vi "DAQ_Analog_Read.vi"(8 "error in (no error)":errorcluster, 11 "task/channels in":refnum<k21>="Photodetectors") -> (0 "error out":errorcluster, 2 "output cluster":T1, 3 "task out":refnum<k21>)   [LabVIEW 2018]
uses:
  SupportVIs/DAQmx Read (Analog 1D DBL NChan 1Samp).vi
  SupportVIs/DAQmx Fill In Error Info.vi
  SupportVIs/NI_PtbyPt.lvlib
panel:
  out "Waveform Chart - Light":T2(graph)
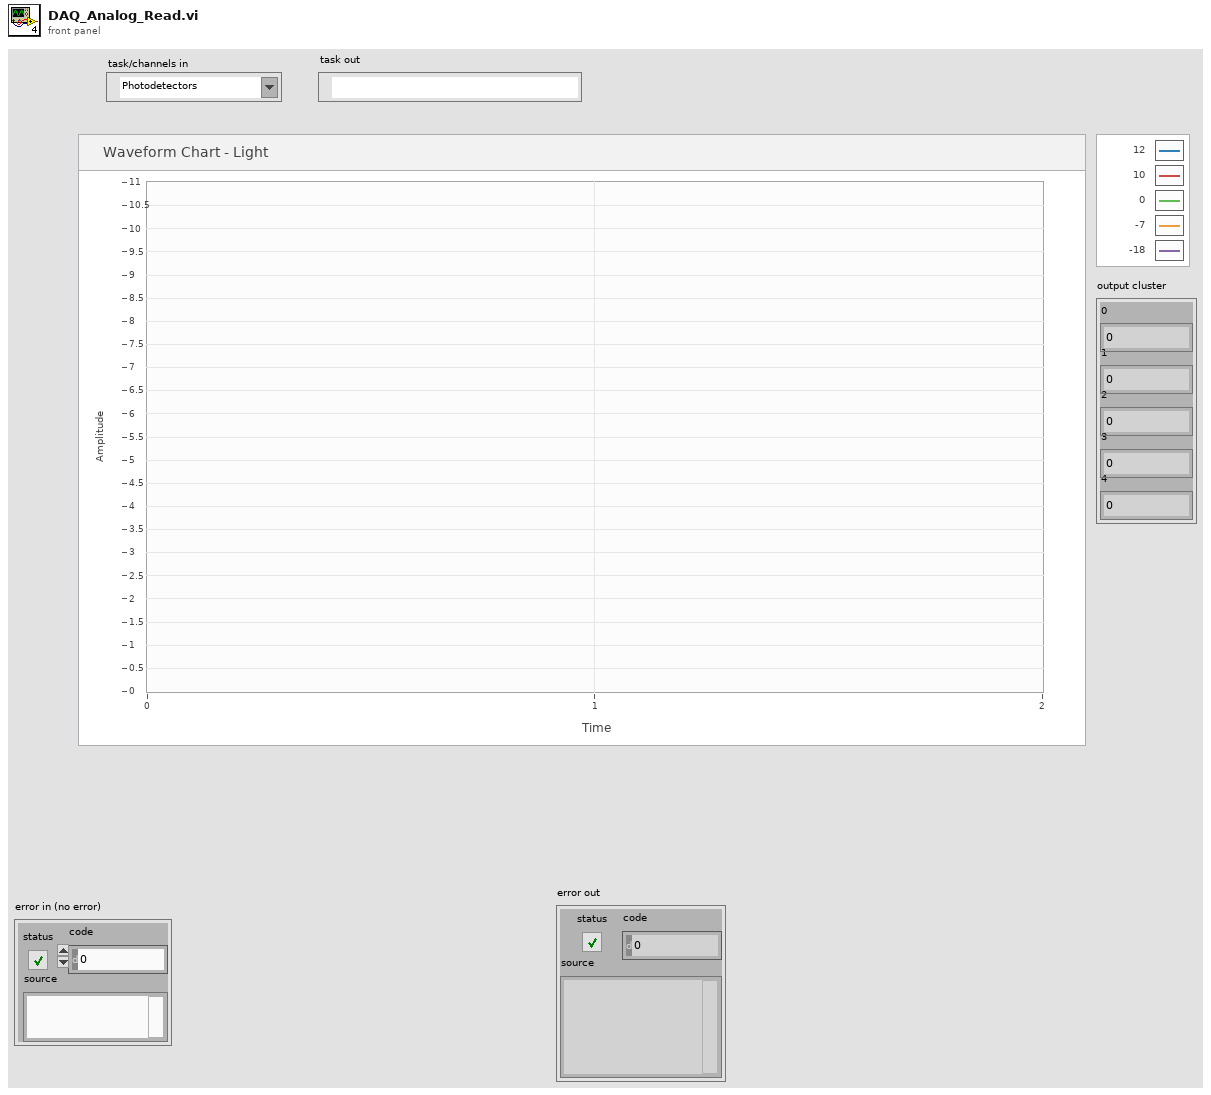
[diagram p1: front panel]
types:
  T1 = cluster{"0":dbl, "1":dbl, "2":dbl, "3":dbl, "4":dbl}
  T2 = cluster{"mean":dbl, "mean":dbl, "mean":dbl, "mean":dbl, "mean":dbl}
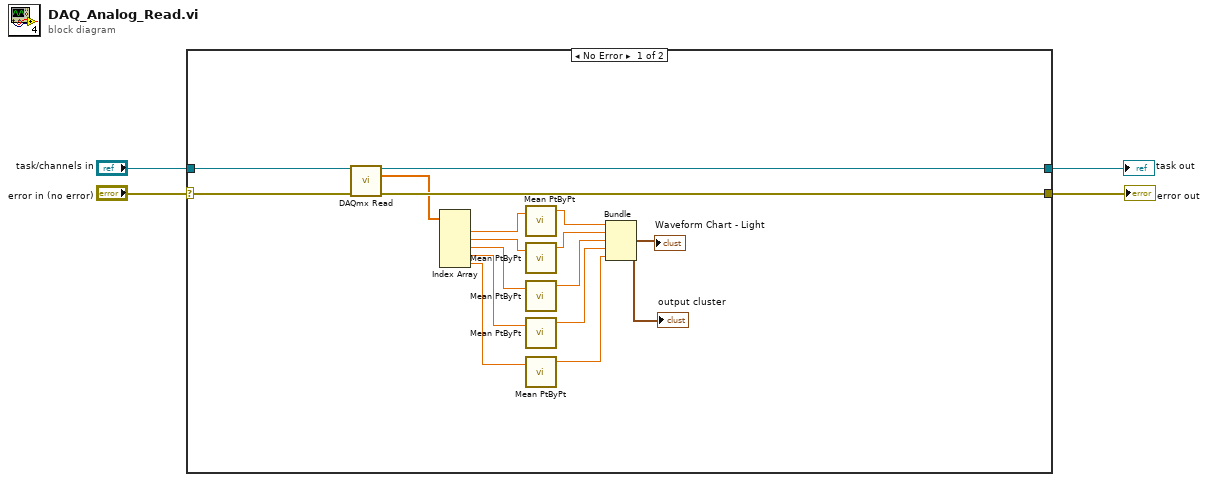
[diagram p0: block diagram]
diagram:
  n1 = case shown="No Error" "error in (no error)" {
    selector: "error in (no error)" -> [w5 w22]
    tunnel: [w20 w22] -> w1
    tunnel: [w19 w21] -> w2
    tunnel: "task/channels in" -> [w6 w21]
    frame No Error {
      n2 = call-poly "DAQmx Read.vi"("task/channels in"=w6, "error in"=w5) -> ("task out"=w19:refnum<k21>, "data"=w18:dbl[], "error out"=w20:errorcluster)  [unwired: 11 in]
      n3 = Index Array(array=w18) -> (element #1=w17:dbl, element #2=w15:dbl, element #3=w12:dbl, element #4=w11:dbl, element #5=w10:dbl)  [unwired: 5 in]
      n4 = call "Mean PtByPt.vi"("x"=w17) -> ("mean"=w16:dbl)  [unwired: 3 in, 1 out]
      n5 = call "Mean PtByPt.vi"("x"=w15) -> ("mean"=w14:dbl)  [unwired: 3 in, 1 out]
      n6 = call "Mean PtByPt.vi"("x"=w12) -> ("mean"=w9:dbl)  [unwired: 3 in, 1 out]
      n7 = call "Mean PtByPt.vi"("x"=w11) -> ("mean"=w8:dbl)  [unwired: 3 in, 1 out]
      n8 = call "Mean PtByPt.vi"("x"=w10) -> ("mean"=w7:dbl)  [unwired: 3 in, 1 out]
      n9 = Bundle("mean"=w16, "mean"=w14, "mean"=w9, "mean"=w8, "mean"=w7) -> (→"Waveform Chart - Light" →"output cluster":T2)  [unwired: 1 in]
    }
    frame Error {
    }
  }
  "error out" <- w1
  "task out" <- w2
